vi "Execute (Return first result with rows).vi"(8 "error in (no error)":errorcluster, 10 "SQL":string, 11 "PQ Connection in":refnum<class "PQ Connection.lvclass">) -> (0 "error out":errorcluster, 1 "First Result with Rows returned":refnum<class "PQ Result.lvclass">, 2 "Number of Rows":i32, 3 "PQ Connection out":refnum<class "PQ Connection.lvclass">)   [LabVIEW 2015, in "PQ Connection.lvclass"]
uses:
  PQ Connection.lvclass
  Result/PQ Result.lvclass
  PQ Connection.lvclass/PQ Connection.ctl
  Result/PQ Result.lvclass/PQ Result.ctl
  libpq.dll
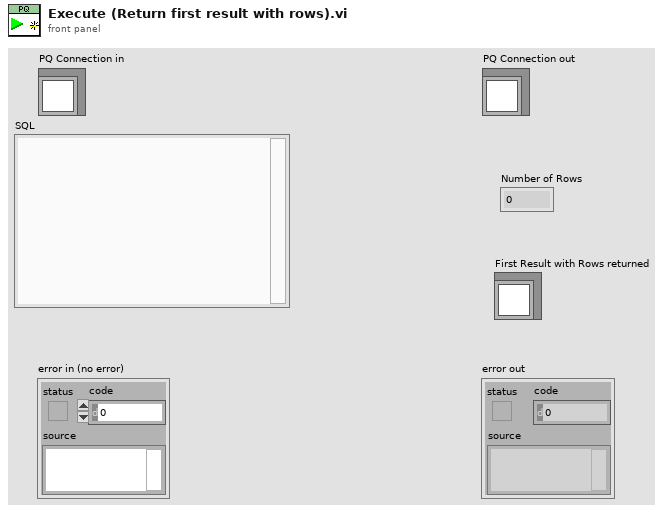
[diagram p1: front panel]
types:
  T1 = typedef "PQ Result.lvclass/Result Status.ctl" = enum32{"PGRES_EMPTY_QUERY", "PGRES_COMMAND_OK", "PGRES_TUPLES_OK", "PGRES_COPY_OUT", "PGRES_COPY_IN", "PGRES_BAD_RESPONSE", "PGRES_NONFATAL_ERROR", "PGRES_FATAL_ERROR", "PGRES_COPY_BOTH", "PGRES_SINGLE_TUPLE"}
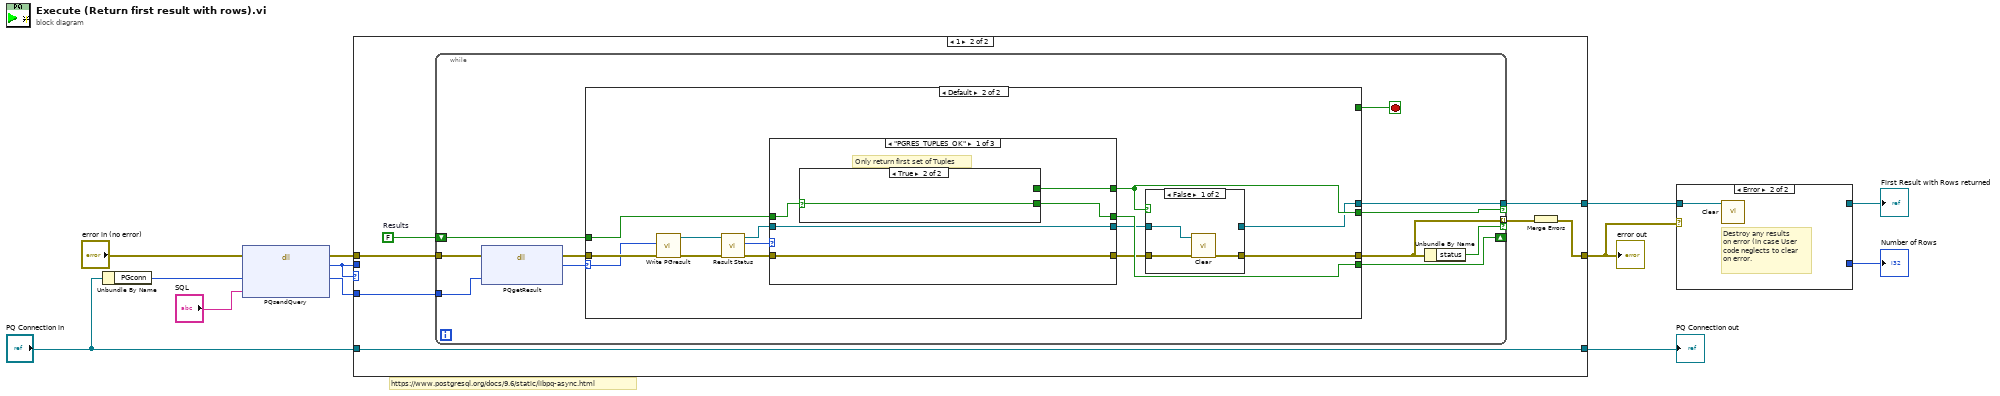
[diagram p0: block diagram]
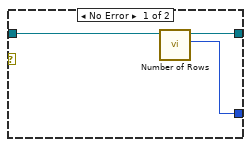
[diagram p2: hidden frame]
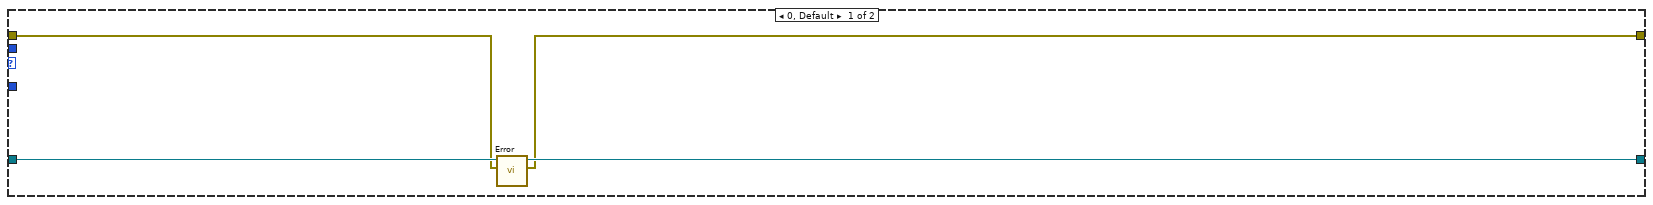
[diagram p3: hidden frame]
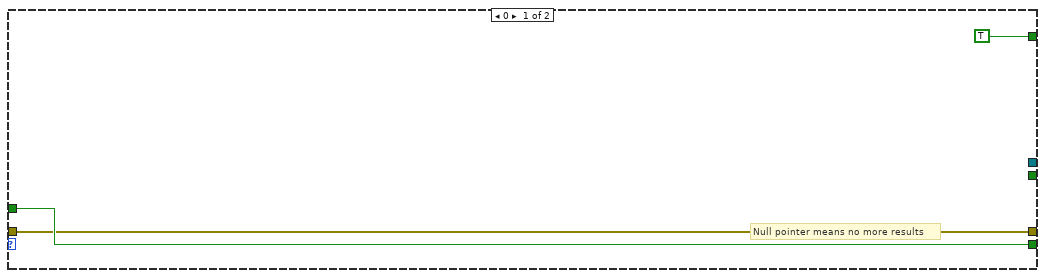
[diagram p4: hidden frame]
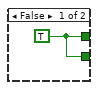
[diagram p5: hidden frame]
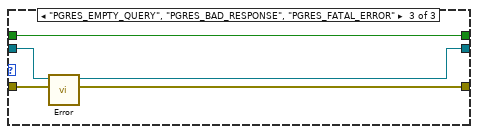
[diagram p7: hidden frame]
diagram:
  # "https://www.postgresql.org/docs/9.6/static/libpq-async.html"
  n1 = Unbundle By Name("PQ Connection in") -> ("PGconn"=w11:u32)
  n2 = dll-call lib="C:/PQ/Connection/libpq.dll" fn="PQsendQuery" ("libpq.*:PQexec")(error in="error in (no error)", "PGconn"=w11, "command"="SQL") -> (error out=w10:errorcluster, "OK?"=w8:u32, "PGconn"=w5:u32)  [unwired: 3 in, 1 out]
  n3 = case shown="1" w8 {
    tunnel: w10 -> [w14 w23]
    tunnel: w8 -> [_ _]
    tunnel: [_ w22] -> w2
    tunnel: [w13 w17] -> w1
    tunnel: "PQ Connection in" -> [w16 w19]
    tunnel: [w15 w19] -> w6
    tunnel: w5 -> [_ w20]
    frame 0, Default {
      n4 = call "Error.vi"("error in (no error)"=w14, "PQ Connection in"=w16) -> ("error out"=w13:errorcluster, "PQ Connection out"=w15:refnum<class "PQ Connection.lvclass">)  [unwired: 8 in]
    }
    frame 1 {
      w18 = FALSE  # Results
      n5 = while {
        tunnel: [w30] -> w22 if=w31
        tunnel: w20 -> [w34]
        shift-right: [w32] -> _
        shift-left: w18 -> [w33]
        tunnel: w23 -> [w27]
        tunnel: [w25] -> w21 mode=indexing if=w24
        stop <- w28 stop-if-true
        n6 = dll-call lib="C:/PQ/Connection/libpq.dll" fn="PQgetResult" ("libpq.*:PQexec")(error in=w27, "PGconn"=w34) -> (error out=w26:errorcluster, "PQresult"=w29:u32)  [unwired: 3 in, 1 out]
        n7 = case shown="Default" w29 {
          selector: w29 -> [_ w38]
          tunnel: w26 -> [w36 w51]
          tunnel: w33 -> [w37 w50]
          tunnel: [w37 w49] -> w32
          tunnel: [_ w48] -> w31
          tunnel: [_ w46] -> w30
          tunnel: [w36 w44] -> w25
          tunnel: [TRUE _] -> w28
          frame 0 {
            # "Null pointer means no more results"
          }
          frame Default {
            n8 = call "Write PGresult.vi"("error in (no error)"=w51, "PGresult"=w38) -> ("error out"=w42:errorcluster, "PQ Result  out"=w43:refnum<class "PQ Result.lvclass">)  [unwired: 8 in]
            n9 = call "Result Status.vi"("error in (no error)"=w42, "PQ Result in"=w43) -> ("error out"=w39:errorcluster, "Result Status"=w41:T1, "PQ Result out"=w40:refnum<class "PQ Result.lvclass">)  [unwired: 7 in]
            n10 = case shown="\"PGRES_TUPLES_OK\"" w41 {
              tunnel: [w55 w59 w62] -> w47
              tunnel: w40 -> [w55 w59 w66]
              tunnel: w39 -> [w56 w61 w65]
              tunnel: [w56 w61 w63] -> w45
              tunnel: [w54 _ _] -> w48
              tunnel: w50 -> [w53 w60 w64]
              tunnel: [w52 w60 w64] -> w49
              frame "PGRES_TUPLES_OK" {
                # "Only return first set of Tuples"
                n11 = case shown="True" w53 {
                  selector: w53 -> [_ w58]
                  tunnel: [w57 _] -> w54
                  tunnel: [w57 w58] -> w52
                  frame False {
                    w57 = TRUE
                  }
                  frame True {
                  }
                }
              }
              frame Default {
                # "No results, but not error"
              }
              frame "PGRES_EMPTY_QUERY", "PGRES_BAD_RESPONSE", "PGRES_FATAL_ERROR" {
                n12 = call "Error.vi"("error in (no error)"=w65, "PQ Result  In"=w66) -> ("error out"=w63:errorcluster, "PQ Result"=w62:refnum<class "PQ Result.lvclass">)  [unwired: 8 in]
              }
            }
            n13 = case shown="False" w48 {
              tunnel: w47 -> [w69 w71]
              tunnel: [_ w71] -> w46
              tunnel: w45 -> [w68 w70]
              tunnel: [w67 w70] -> w44
              frame False {
                n14 = call "Clear.vi"("error in (no error)"=w68, "PQ Result  in"=w69) -> ("error out"=w67:errorcluster)  [unwired: 9 in]
              }
              frame True {
              }
            }
          }
        }
        n15 = Unbundle By Name(w25) -> ("status"=w24:bool)
      }
      n16 = Merge Errors(w21) -> (w17:errorcluster)
    }
  }
  "error out" <- w1
  "PQ Connection out" <- w6
  n17 = case shown="Error" w1 {
    tunnel: [w74 _] -> w4
    tunnel: [w73 _] -> w3
    tunnel: w2 -> [w72 w75]
    frame No Error {
      n18 = call "Number of Rows.vi"("PQ Result in"=w72) -> ("Number of Rows"=w74:i32, "PQ Result out"=w73:refnum<class "PQ Result.lvclass">)  [unwired: 8 in, 1 out]
    }
    frame Error {
      # "Destroy any results\non error (in case User\ncode neglects to clear\non error."
      n19 = call "Clear.vi"("PQ Result  in"=w75) -> ()  [unwired: 10 in, 1 out]
    }
  }
  "First Result with Rows returned" <- w3
  "Number of Rows" <- w4
